vi "ROIed Video Frame Create.vi"(4 "Apply? (T)":bool=TRUE, 5 "Depth Scale":dbl, 6 "ROI Descriptor":T3 {"Contours"."Type" items=["No Selection", "Point", "Line", "Rectangle", "Oval", "Polygon", "Freehand Region", "Annulus", "Unused2", "Unused3", "Broken Line", "Freehand Line", "Rotated Rectangle"]}, 7 "Frame Number":i32, 8 "error in (no error)":errorcluster, 9 "Frame Data":T1, 10 "Image Dst":T2, 11 "ROIed Video Frame in":refnum<class "ROIed Video Frame.lvclass">) -> (0 "error out":errorcluster, 3 "ROIed Video Frame out":refnum<class "ROIed Video Frame.lvclass">)   [LabVIEW 2018, in "ROIed Video Frame.lvclass"]
uses:
  ROIed Video Frame.lvclass
  C:/Users/aaron.jencks/Documents/GitHub/emerson_seed_object_detection/LabVIEW/Projects/Paul's Video Viewer/Classes/Video Frame/Video Frame.lvclass
  <vilib>/vision/Image Controls.llb/IMAQ Image.ctl
  ROIed Video Frame.lvclass/ROIed Video Frame.ctl
  Video Frame/Video Frame.lvclass
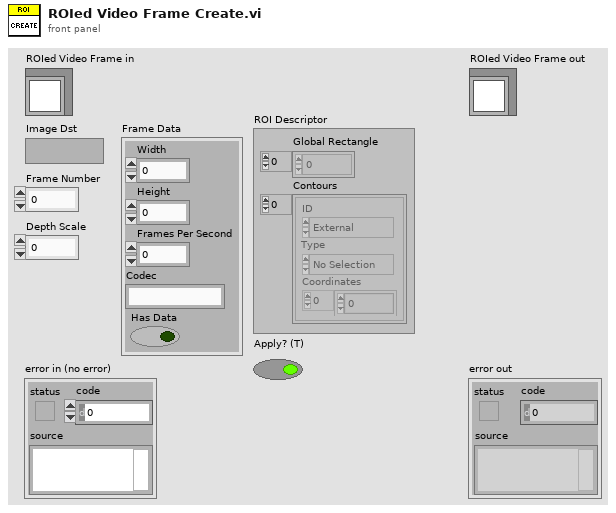
[diagram p1: front panel]
types:
  T1 = cluster{"Width":u32, "Height":u32, "Frames Per Second":u32, "Codec":string, "Has Data":bool}
  T2 = typedef "IMAQ Image.ctl" = refnum<image>
  T3 = typedef "ROI Descriptor" = cluster{"Global Rectangle":i32[], "Contours":cluster{"ID":enum32{"External", "Internal"}, "Type":u32, "Coordinates":i32[]}[]}
  T4 = typedef "Image Type" = u32
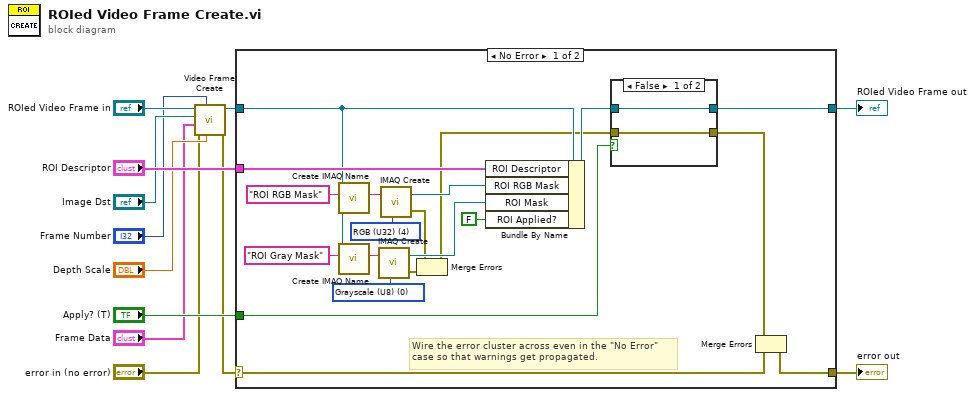
[diagram p0: block diagram]
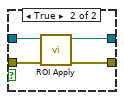
[diagram p2: hidden frame]
diagram:
  n1 = call "Video Frame Create.vi"("Depth Scale"="Depth Scale", "Frame Number"="Frame Number", "error in (no error)"="error in (no error)", "Frame Data"="Frame Data", "Image Dst"="Image Dst", "Video Frame in"="ROIed Video Frame in") -> ("error out"=w1:errorcluster, "Video Frame out"=w7:refnum<class "ROIed Video Frame.lvclass">)  [unwired: 4 in]
  n2 = case shown="No Error" w1 {
    selector: w1 -> [w15 w40]
    tunnel: [w13 w40] -> w12
    tunnel: [w20 w39] -> w11
    tunnel: w7 -> [w26 w39]
    tunnel: "ROI Descriptor" -> [w32 _]
    tunnel: "Apply? (T)" -> [w19 _]
    frame No Error {
      w25 = T4 0 items=["Grayscale (U8)", "Grayscale (I16)", "Grayscale (SGL)", "Complex (CSG)", "RGB (U32)", "HSL (U32)", "RGB (U64)", "Grayscale (U16)"] ("Image Type")
      w29 = T4 4 items=["Grayscale (U8)", "Grayscale (I16)", "Grayscale (SGL)", "Complex (CSG)", "RGB (U32)", "HSL (U32)", "RGB (U64)", "Grayscale (U16)"] ("Image Type")
      # "Wire the error cluster across even in the \"No Error\"\ncase so that warnings get propagated."
      n3 = call-dynamic "Create IMAQ Name.vi"("Name (\"\")"="ROI RGB Mask" ("Name (\"\")"), "Video Frame in"=w26) -> ("Name Out"=w30:string)  [unwired: 7 in, 2 out]
      n4 = call-dynamic "Create IMAQ Name.vi"("Name (\"\")"="ROI Gray Mask" ("Name (\"\")"), "Video Frame in"=w26) -> ("Name Out"=w27:string)  [unwired: 7 in, 2 out]
      n5 = call "IMAQ Create"("Image Name"=w27, "Image Type"=w25) -> ("New Image"=w22:T2, "error out"=w17:errorcluster)  [unwired: 3 in]
      n6 = call "IMAQ Create"("Image Name"=w30, "Image Type"=w29) -> ("New Image"=w28:T2, "error out"=w18:errorcluster)  [unwired: 3 in]
      n7 = Merge Errors(w18, w17) -> (w16:errorcluster)
      n8 = Bundle By Name(cluster=w26, "ROI Descriptor"=w32, "ROI RGB Mask"=w28, "ROI Mask"=w22, "ROI Applied?"=FALSE) -> (w21:refnum<class "ROIed Video Frame.lvclass">)
      n9 = case shown="False" w19 {
        tunnel: w21 -> [w34 w38]
        tunnel: [w34 w37] -> w20
        tunnel: w16 -> [w33 w36]
        tunnel: [w33 w35] -> w14
        frame False {
        }
        frame True {
          n10 = call-dynamic "ROI Apply.vi"("error in (no error)"=w36, "ROIed Video Frame in"=w38) -> ("error out"=w35:errorcluster, "ROIed Video Frame out"=w37:refnum<class "ROIed Video Frame.lvclass">)  [unwired: 8 in]
        }
      }
      n11 = Merge Errors(w14, w15) -> (w13:errorcluster)
    }
    frame Error {
    }
  }
  "error out" <- w12
  "ROIed Video Frame out" <- w11
